vi "spancheckdata.vi"(0 "object in":refnum<class "212format_work.lvclass">, 1 "in":T2, 5 "error in (no error)":errorcluster) -> (14 "object out":refnum<class "212format_work.lvclass">, 15 "out":T1, 19 "error out":errorcluster)   [LabVIEW 2016, in "212format_work.lvclass"]
uses:
  212format_work.lvclass
  212format_work.lvclass/212format_work.ctl
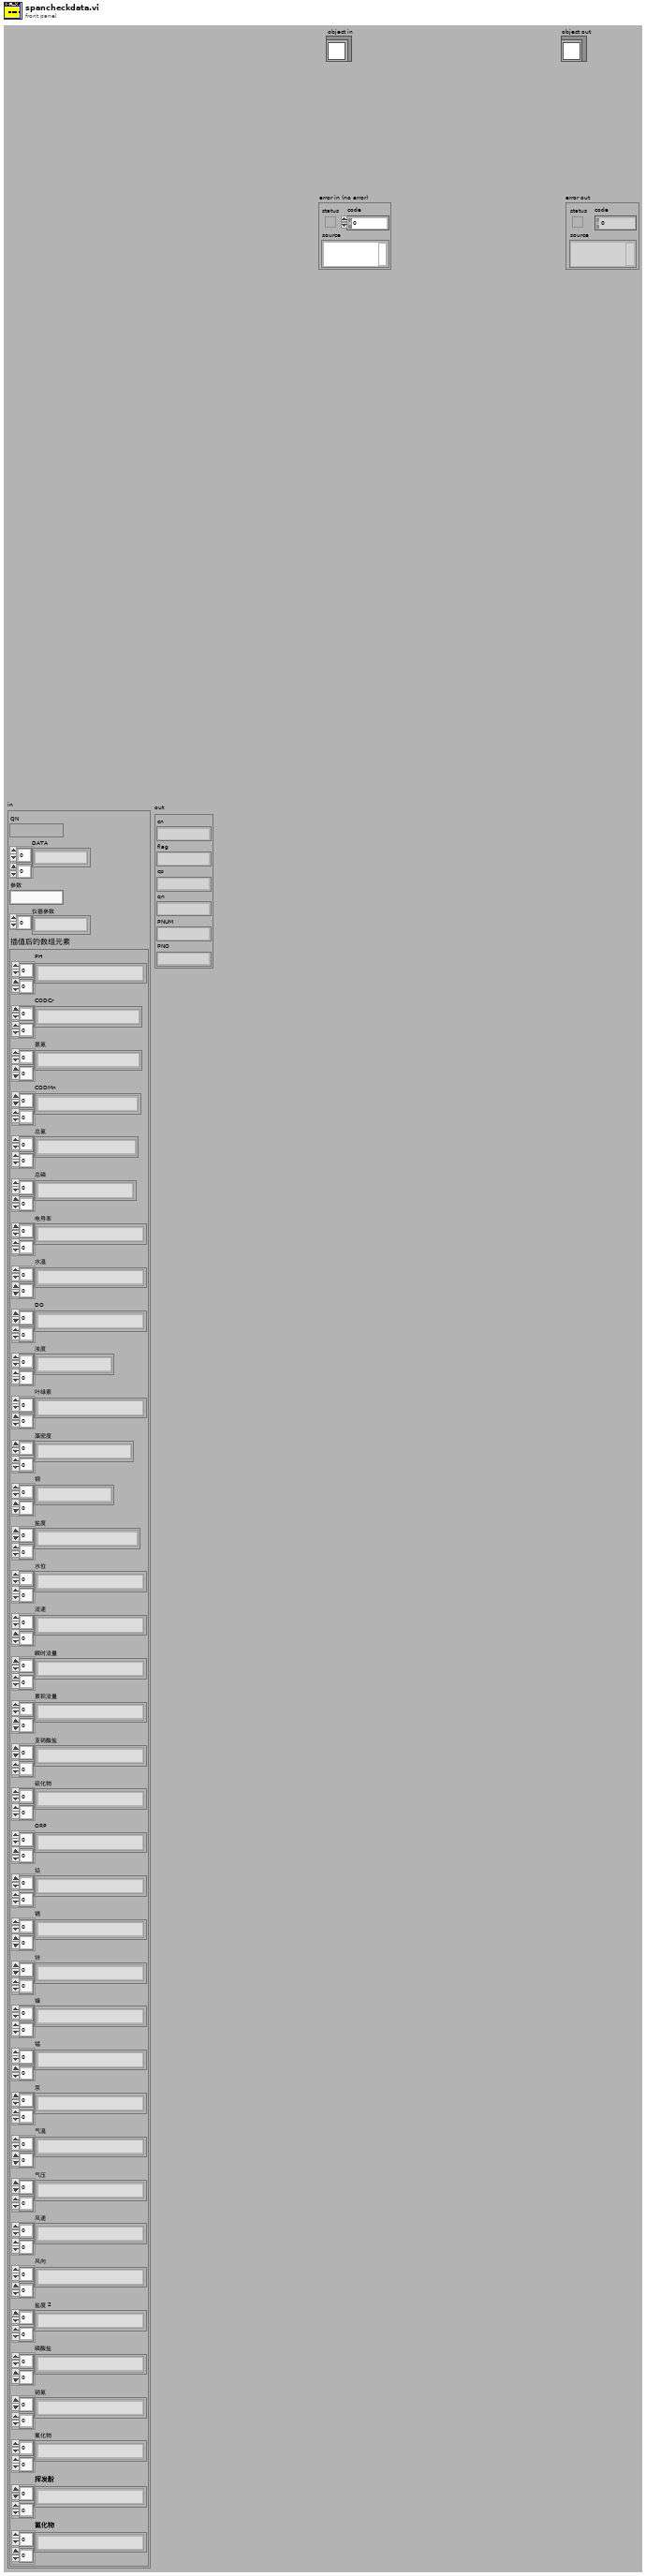
[diagram p1: front panel]
types:
  T1 = cluster{"cn":string, "flag":string, "cp":string, "qn":string, "PNUM":string, "PNO":string}
  T2 = cluster{"QN":string, "DATA":string[][], "参数":string, "仪器参数":string[], "插值后的数组元素":cluster{"PH":string[][], "CODCr":string[][], "氨氮":string[][], "CODMn":string[][], "总氮":string[][], "总磷":string[][], "电导率":string[][], "水温":string[][], "DO":string[][], "浊度":string[][], "叶绿素":string[][], "藻密度":string[][], "铜":string[][], "盐度":string[][], "水位":string[][], "流速":string[][], "瞬时流量":string[][], "累积流量":string[][], "亚硝酸盐":string[][], "硫化物":string[][], "ORP":string[][], "铅":string[][], "镉":string[][], "锌":string[][], "镍":string[][], "锰":string[][], "汞":string[][], "气温":string[][], "气压":string[][], "风速":string[][], "风向":string[][], "盐度 2":string[][], "磷酸盐":string[][], "硝氮":string[][], "氟化物":string[][], "挥发酚":string[][], "氯化物":string[][]}}
  T3 = enum16{"小时数据", "实时数据", "平行样测试", "集成干预测试", "加标回收测试", "核查数据", "空白零点跨度数据", "提取小时数据", "提取实时数据", "操作日志", "仪器参数", "3090仪器参数", "提取仪器参数", "报警信息"}
  T4 = typedef "212format_work.lvclass/interdata控件.ctl" = cluster{"数据发送协议":enum16{"2005-212协议", "2017-212协议"}, "枚举":enum16{"返回请求应答", "上传数据", "返回执行结果"}, "系统编码ST":string, "主动上报数据中":bool, "数据组合发送":bool, "地表水/污染源":bool, "应用环境":enum16{"STD", "GB212"}}
  T5 = typedef "212format_work.lvclass/data控件.ctl" = cluster{"选择发送的参数":string, "插值后的数组元素":cluster{"PH":string[][], "CODCr":string[][], "氨氮":string[][], "CODMn":string[][], "总氮":string[][], "总磷":string[][], "电导率":string[][], "水温":string[][], "DO":string[][], "浊度":string[][], "叶绿素":string[][], "藻密度":string[][], "铜":string[][], "盐度":string[][], "水位":string[][], "流速":string[][], "瞬时流量":string[][], "累积流量":string[][], "亚硝酸盐":string[][], "硫化物":string[][], "ORP":string[][], "铅":string[][], "镉":string[][], "锌":string[][], "镍":string[][], "锰":string[][], "汞":string[][], "气温":string[][], "气压":string[][], "风速":string[][], "风向":string[][], "盐度 2":string[][], "磷酸盐":string[][], "硝氮":string[][], "氟化物":string[][], "挥发酚":string[][], "氯化物":string[][]}, "register values":u16[], "columns输出":string[], "环境参数":string[][], "仪器编码":string, "实时数据发送间隔":u32, "实时数据参数":string, "参数系数簇":cluster{"CODMn":dbl, "CODCr":dbl, "DO":dbl, "铜":dbl, "PH":dbl, "氨氮":dbl, "比电导率":dbl, "水温":dbl, "COD":dbl, "浊度":dbl, "总氮":dbl, "总磷":dbl, "叶绿素a":dbl, "藻密度":dbl, "水位":dbl, "流速":dbl, "瞬时流量":dbl, "累积流量":dbl, "亚硝酸盐":dbl, "硫化物":dbl, "ORP":dbl, "铅":dbl, "镉":dbl, "锌":dbl, "镍":dbl, "锰":dbl, "汞":dbl, "气温":dbl, "气压":dbl, "风速":dbl, "风向":dbl, "盐度":dbl, "磷酸盐":dbl, "硝氮":dbl, "氟化物":dbl, "挥发酚":dbl, "氯化物":dbl}, "因子编码簇":cluster{"CODMn":string, "CODCr":string, "DO":string, "铜":string, "PH":string, "氨氮":string, "比电导率":string, "水温":string, "COD":string, "浊度":string, "总氮":string, "总磷":string, "叶绿素a":string, "藻密度":string, "水位":string, "流速":string, "瞬时流量":string, "累积流量":string, "亚硝酸盐":string, "硫化物":string, "ORP":string, "铅":string, "镉":string, "锌":string, "镍":string, "锰":string, "汞":string, "气温":string, "气压":string, "风速":string, "风向":string, "盐度":string, "磷酸盐":string, "硝氮":string, "氟化物":string, "挥发酚":string, "氯化物":string}, "小时数据发送次数":i32, "读取试剂余量的值":u16[], "参数编码":string, "数据数组大小":i32, "总包数":i32, "当前包号":i32, "columns":string[], "剖面多参数":string[][], "分包标准":i32}
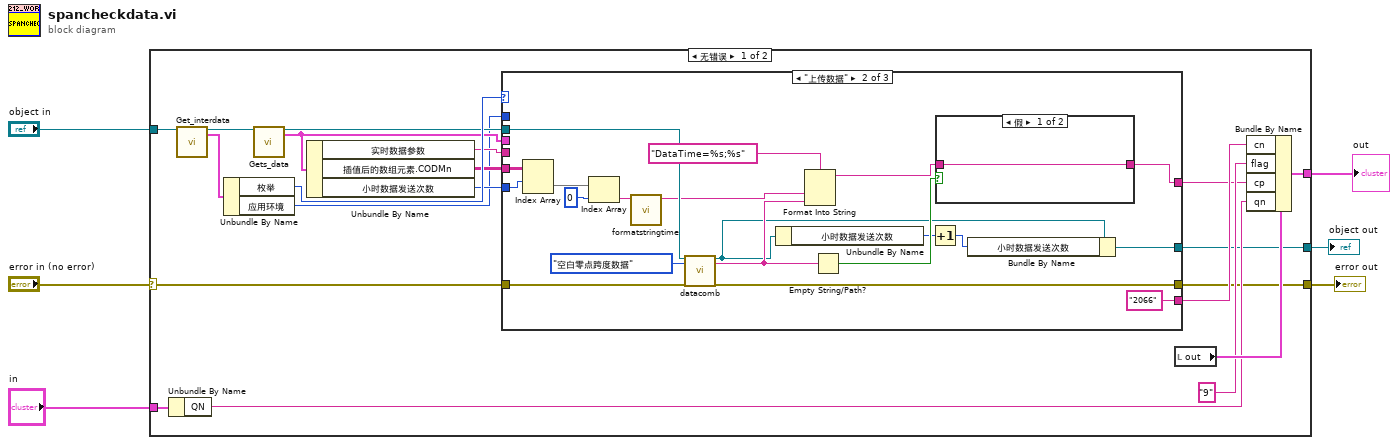
[diagram p0: block diagram]
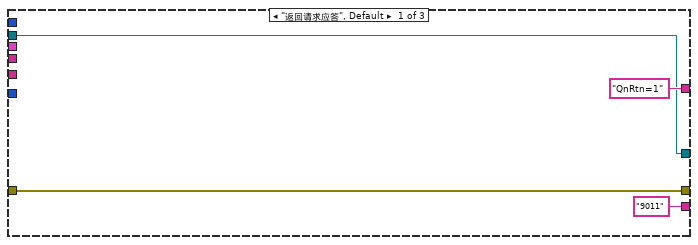
[diagram p2: hidden frame]
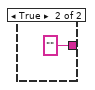
[diagram p3: hidden frame]
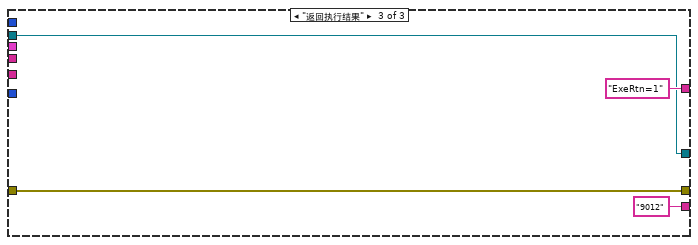
[diagram p4: hidden frame]
diagram:
  n1 = case shown="无错误" "error in (no error)" {
    selector: "error in (no error)" -> [w24 w58]
    tunnel: [w7 w58] -> w5
    tunnel: [w8 w57] -> w3
    tunnel: "object in" -> [w25 w57]
    tunnel: "in" -> [w26 _]
    tunnel: [w9 _] -> w1
    frame No Error {
      n2 = Unbundle By Name(w26) -> ("QN"=w19:string)
      n3 = call-dynamic "Get_interdata.vi"("object in"=w25) -> ("object out"=w16:refnum<class "212format_work.lvclass">, "interdata"=w18:T4)  [unwired: 16 in, 1 out]
      n4 = Unbundle By Name(w18) -> ("枚举"=w17:enum16{"返回请求应答", "上传数据", "返回执行结果"}, "应用环境"=w10:enum16{"STD", "GB212"})
      n5 = call-dynamic "Gets_data.vi"("object in"=w16) -> ("object out"=w14:refnum<class "212format_work.lvclass">, "data"=w11:T5)  [unwired: 16 in, 1 out]
      n6 = Unbundle By Name(w11) -> ("实时数据参数"=w15:string, "插值后的数组元素.CODMn"=w13:string[][], "小时数据发送次数"=w12:i32)
      n7 = case shown="\"上传数据\"" w17 {
        tunnel: ["9011" ("CN") "2066" ("CN") "9012" ("CN")] -> w22
        tunnel: ["QnRtn=1" w49 "ExeRtn=1"] -> w20
        tunnel: w15 -> [_ _ _]
        tunnel: w14 -> [w28 w50 w53]
        tunnel: [w28 w33 w53] -> w8
        tunnel: w24 -> [w27 w48 w54]
        tunnel: [w27 w47 w54] -> w7
        tunnel: w13 -> [_ w46 _]
        tunnel: w12 -> [_ w45 _]
        tunnel: w11 -> [_ _ _]
        tunnel: w10 -> [_ _ _]
        frame "返回请求应答", Default {
        }
        frame "上传数据" {
          n8 = Index Array(array=w46, index (row)=w45) -> (element=w43:string[])  [unwired: 1 in]
          n9 = Index Array(array=w43, index=0 ("索引")) -> (element=w41:string)
          n10 = call "formatstringtime.vi"("字符串"=w41) -> ("result string"=w38:string)  [unwired: 10 in]
          n11 = call-dynamic "datacomb.vi"("object in"=w50, "枚举"=T3."空白零点跨度数据", "error in (no error)"=w48) -> ("object out"=w32:refnum<class "212format_work.lvclass">, "字符串"=w37:string, "error out"=w47:errorcluster)  [unwired: 14 in]
          n12 = Unbundle By Name(w32) -> ("小时数据发送次数"=w35:i32)
          n13 = Format Into String(format string="DataTime=%s;%s", w38, w37) -> (resulting string=w36:string)  [unwired: 2 in, 1 out]
          n14 = Empty String/Path?(string/path=w37) -> (empty?=w39:bool)
          n15 = Increment(x=w35) -> (x+1=w34:i32)
          n16 = case shown="假" w39 {
            tunnel: [w51 ""] -> w49
            tunnel: w36 -> [w51 _]
            frame False {
            }
            frame True {
            }
          }
          n17 = Bundle By Name(cluster=w32, "小时数据发送次数"=w34) -> (w33:refnum<class "212format_work.lvclass">)
        }
        frame "返回执行结果" {
        }
      }
      n18 = local read "out"() -> (w23:T1)
      n19 = Bundle By Name(cluster=w23, "cn"=w22, "flag"="9" ("ST"), "cp"=w20, "qn"=w19) -> (w9:T1)
    }
    frame Error {
    }
  }
  "error out" <- w5
  "object out" <- w3
  "out" <- w1
